vi "例11.7Demo-Main.vi"() -> ()   [LabVIEW 2015]
panel:
  out "BufferSize out":i32
  out "Error out":errorcluster
  in  "stop":bool
  out "Waveform Chart":dbl[](graph)
  out "szDeviceName":string
  out "szSN":string
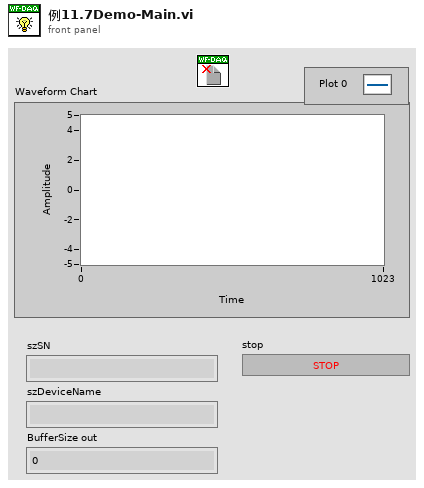
[diagram p1: front panel]
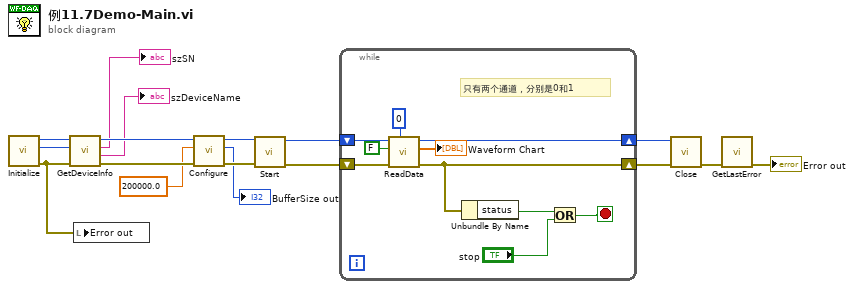
[diagram p0: block diagram]
diagram:
  n1 = call <vilib>:"Initialize.vi"() -> ("error out"=w1:errorcluster, "idxDevice out"=w16:i32, "instrumentHandle out"=w17:i32)  [unwired: 9 in]
  n2 = call <vilib>:"GetDeviceInfo.vi"("Error in"=w1, "idxDevice"=w16, "instrumentHandle in"=w17) -> ("Error out"=w14:errorcluster, "szDeviceName"=→"szDeviceName":string, "szSN"=→"szSN":string, "instrumentHandle out"=w15:i32)  [unwired: 5 in]
  n3 = local write "Error out"(w1) -> ()
  n4 = call <vilib>:"Configure.vi"("Error in"=w14, "hzFrequency(1000)"=200000.0, "instrumentHandle in"=w15) -> ("Error out"=w12:errorcluster, "BufferSize out"=→"BufferSize out":i32, "instrumentHandle out"=w13:i32)  [unwired: 6 in]
  n5 = call <vilib>:"Start.vi"("Error in"=w12, "instrumentHandle in"=w13) -> ("Error out"=w3:errorcluster, "instrumentHandle out"=w2:i32)  [unwired: 8 in]
  n6 = while {
    shift-right: [w23] -> w10
    shift-left: w3 -> [w27]
    shift-right: [w25] -> w11
    shift-left: w2 -> [w26]
    stop <- w20 stop-if-true
    # "只有两个通道，分别是0和1"
    n7 = call <vilib>:"ReadData.vi"("idxChannel"=0, "Error in"=w27, "Enable DAQ Lost Error(True)"=FALSE, "instrumentHandle in"=w26) -> ("Error out"=w23:errorcluster, "Waveform Chart"=→"Waveform Chart":dbl[], "instrumentHandle out"=w25:i32)  [unwired: 4 in, 1 out]
    n8 = Unbundle By Name(w23) -> ("status"=w22:bool)
    n9 = Or(x=w22, y="stop") -> (x .or. y?=w20:bool)
  }
  n10 = call <vilib>:"Close.vi"("Error in"=w10, "instrumentHandle in"=w11) -> ("Error out"=w9:errorcluster)  [unwired: 9 in]
  n11 = call <vilib>:"GetLastError.vi"("Error in"=w9) -> ("Error out"=→"Error out":errorcluster)  [unwired: 10 in]
